vi "Lab Panel V5.26.vi"() -> ()   [LabVIEW 2017] (continued)
              tunnel: w3351 -> [w3361 _ w3422]
              tunnel: w3350 -> [w3359 _ w3421]
              tunnel: w3349 -> [w3360 _ w3420]
              tunnel: w3348 -> [_ w3384 w3419]
              tunnel: w3347 -> [_ w3385 w3418]
              tunnel: w3346 -> [_ w3386 w3417]
              tunnel: w3345 -> [_ w3387 w3416]
              tunnel: w3344 -> [_ w3388 w3415]
              frame #0 {
                n1780 = Select(t=2, s=w3359, f=0) -> (s? t:f=w3355:i32)
                n1781 = Select(t=2, s=w3361, f=0) -> (s? t:f=w3356:i32)
                n1782 = Select(t=2, s=w3360, f=0) -> (s? t:f=w3354:i32)
                n1783 = Select(t=2, s=w3367, f=0) -> (s? t:f=w3358:i32)
                n1784 = Select(t=2, s=w3362, f=0) -> (s? t:f=w3357:i32)
                n1785 = property on="SELECT LAB02-2" class="RadioBtnsControl (strict)"("DisabledEnum"=w3355) -> ()  [unwired: 2 in, 2 out]
                n1786 = property on="SELECT LAB02-1" class="RadioBtnsControl (strict)"("DisabledEnum"=w3356) -> ()  [unwired: 2 in, 2 out]
                n1787 = property on="SELECT LAB03-1" class="RadioBtnsControl (strict)"("DisabledEnum"=w3354) -> ()  [unwired: 2 in, 2 out]
                n1788 = property on="SELECT LAB01-1" class="RadioBtnsControl (strict)"("DisabledEnum"=w3358) -> ()  [unwired: 2 in, 2 out]
                n1789 = property on="SELECT LAB01-2" class="RadioBtnsControl (strict)"("DisabledEnum"=w3357) -> ()  [unwired: 2 in, 2 out]
                n1790 = Not(x=w3367) -> (.not. x?=w3368:bool)
                n1791 = property on="RESULT LAB01-1" class="Bool (strict)"("Visible"=w3368) -> ()  [unwired: 2 in, 2 out]
                n1792 = Not(x=w3362) -> (.not. x?=w3366:bool)
                n1793 = Not(x=w3361) -> (.not. x?=w3365:bool)
                n1794 = Not(x=w3359) -> (.not. x?=w3364:bool)
                n1795 = property on="RESULT LAB01-2" class="Bool (strict)"("Visible"=w3366) -> ()  [unwired: 2 in, 2 out]
                n1796 = Not(x=w3360) -> (.not. x?=w3363:bool)
                n1797 = property on="RESULT LAB02-1" class="Bool (strict)"("Visible"=w3365) -> ()  [unwired: 2 in, 2 out]
                n1798 = property on="RESULT LAB02-2" class="Bool (strict)"("Visible"=w3364) -> ()  [unwired: 2 in, 2 out]
                n1799 = property on="RESULT LAB03-1" class="Bool (strict)"("Visible"=w3363) -> ()  [unwired: 2 in, 2 out]
                n1800 = property on="SET LAB01-1" class="Clust (strict)"("DisabledEnum"=w3358) -> ()  [unwired: 2 in, 2 out]
                n1801 = property on="SET LAB01-2" class="Clust (strict)"("DisabledEnum"=w3357) -> ()  [unwired: 2 in, 2 out]
                n1802 = property on="SET LAB02-1" class="Clust (strict)"("DisabledEnum"=w3356) -> ()  [unwired: 2 in, 2 out]
                n1803 = property on="SET LAB02-2" class="Clust (strict)"("DisabledEnum"=w3355) -> ()  [unwired: 2 in, 2 out]
                n1804 = property on="SET LAB03-1" class="Clust (strict)"("DisabledEnum"=w3354) -> ()  [unwired: 2 in, 2 out]
                n1805 = property on="O/I  LAB01-1" class="Bool (strict)"("DisabledEnum"=w3358) -> ()  [unwired: 2 in, 2 out]
                n1806 = property on="O/I  LAB01-2" class="Bool (strict)"("DisabledEnum"=w3357) -> ()  [unwired: 2 in, 2 out]
                n1807 = property on="O/I  LAB02-1" class="Bool (strict)"("DisabledEnum"=w3356) -> ()  [unwired: 2 in, 2 out]
                n1808 = property on="O/I  LAB02-2" class="Bool (strict)"("DisabledEnum"=w3355) -> ()  [unwired: 2 in, 2 out]
                n1809 = property on="O/I  LAB03-1" class="Bool (strict)"("DisabledEnum"=w3354) -> ()  [unwired: 2 in, 2 out]
              }
              frame #1 {
                n1810 = Select(t=2, s=w3388, f=0) -> (s? t:f=w3379:i32)
                n1811 = Select(t=2, s=w3387, f=0) -> (s? t:f=w3380:i32)
                n1812 = Select(t=2, s=w3384, f=0) -> (s? t:f=w3383:i32)
                n1813 = Select(t=2, s=w3385, f=0) -> (s? t:f=w3382:i32)
                n1814 = Select(t=2, s=w3386, f=0) -> (s? t:f=w3381:i32)
                n1815 = property on="SELECT LAB05-2" class="RadioBtnsControl (strict)"("DisabledEnum"=w3379) -> ()  [unwired: 2 in, 2 out]
                n1816 = property on="SELECT LAB05-1" class="RadioBtnsControl (strict)"("DisabledEnum"=w3380) -> ()  [unwired: 2 in, 2 out]
                n1817 = property on="SELECT LAB03-2" class="RadioBtnsControl (strict)"("DisabledEnum"=w3383) -> ()  [unwired: 2 in, 2 out]
                n1818 = property on="SELECT LAB04-1" class="RadioBtnsControl (strict)"("DisabledEnum"=w3382) -> ()  [unwired: 2 in, 2 out]
                n1819 = property on="SELECT LAB04-2" class="RadioBtnsControl (strict)"("DisabledEnum"=w3381) -> ()  [unwired: 2 in, 2 out]
                n1820 = property on="SET LAB05-2" class="Clust (strict)"("DisabledEnum"=w3379) -> ()  [unwired: 2 in, 2 out]
                n1821 = property on="SET LAB05-1" class="Clust (strict)"("DisabledEnum"=w3380) -> ()  [unwired: 2 in, 2 out]
                n1822 = property on="SET LAB03-2" class="Clust (strict)"("DisabledEnum"=w3383) -> ()  [unwired: 2 in, 2 out]
                n1823 = property on="SET LAB04-1" class="Clust (strict)"("DisabledEnum"=w3382) -> ()  [unwired: 2 in, 2 out]
                n1824 = property on="SET LAB04-2" class="Clust (strict)"("DisabledEnum"=w3381) -> ()  [unwired: 2 in, 2 out]
                n1825 = property on="O/I  LAB05-2" class="Bool (strict)"("DisabledEnum"=w3379) -> ()  [unwired: 2 in, 2 out]
                n1826 = property on="O/I  LAB05-1" class="Bool (strict)"("DisabledEnum"=w3380) -> ()  [unwired: 2 in, 2 out]
                n1827 = property on="O/I  LAB04-1" class="Bool (strict)"("DisabledEnum"=w3382) -> ()  [unwired: 2 in, 2 out]
                n1828 = property on="O/I  LAB04-2" class="Bool (strict)"("DisabledEnum"=w3381) -> ()  [unwired: 2 in, 2 out]
                n1829 = property on="O/I  LAB03-2" class="Bool (strict)"("DisabledEnum"=w3383) -> ()  [unwired: 2 in, 2 out]
                n1830 = Not(x=w3388) -> (.not. x?=w3389:bool)
                n1831 = Not(x=w3387) -> (.not. x?=w3390:bool)
                n1832 = Not(x=w3386) -> (.not. x?=w3391:bool)
                n1833 = property on="RESULT LAB05-2" class="Bool (strict)"("Visible"=w3389) -> ()  [unwired: 2 in, 2 out]
                n1834 = property on="RESULT LAB05-1" class="Bool (strict)"("Visible"=w3390) -> ()  [unwired: 2 in, 2 out]
                n1835 = Not(x=w3385) -> (.not. x?=w3392:bool)
                n1836 = property on="RESULT LAB04-2" class="Bool (strict)"("Visible"=w3391) -> ()  [unwired: 2 in, 2 out]
                n1837 = Not(x=w3384) -> (.not. x?=w3393:bool)
                n1838 = property on="RESULT LAB04-1" class="Bool (strict)"("Visible"=w3392) -> ()  [unwired: 2 in, 2 out]
                n1839 = property on="RESULT LAB03-2" class="Bool (strict)"("Visible"=w3393) -> ()  [unwired: 2 in, 2 out]
              }
              frame #2 {
                # "disable calibrate if any test running"
                n1840 = Or(x=w3416, y=w3415) -> (x .or. y?=w3409:bool)
                n1841 = Or(x=w3418, y=w3417) -> (x .or. y?=w3411:bool)
                n1842 = Or(x=w3422, y=w3421) -> (x .or. y?=w3413:bool)
                n1843 = Or(x=w3420, y=w3419) -> (x .or. y?=w3412:bool)
                n1844 = Or(x=w3424, y=w3423) -> (x .or. y?=w3414:bool)
                n1845 = Or(x=w3412, y=w3411) -> (x .or. y?=w3410:bool)
                n1846 = Or(x=w3414, y=w3413) -> (x .or. y?=w3408:bool)
                n1847 = Or(x=w3410, y=w3409) -> (x .or. y?=w3407:bool)
                n1848 = Or(x=w3408, y=w3407) -> (x .or. y?=w3404:bool)
                "Any Test Running" <- w3404
                n1849 = case shown="False" w3404 {
                  tunnel: [0 2] -> w3406
                  frame False {
                  }
                  frame True {
                  }
                }
                n1850 = property on="JIG TEST" class="Clust (strict)"("DisabledEnum"=w3406) -> ()  [unwired: 2 in, 2 out]
                n1851 = property on="Network Directory" class="Path"("DisabledEnum"=w3406) -> ()  [unwired: 2 in, 2 out]
                n1852 = property on="MAIL SETTINGS" class="Clust (strict)"("DisabledEnum"=w3406) -> ()  [unwired: 2 in, 2 out]
                n1853 = property on="SET (cal)" class="Bool (strict)"("DisabledEnum"=w3406) -> ()  [unwired: 2 in, 2 out]
                n1854 = property on="ADMIN" class="Bool (strict)"("DisabledEnum"=0) -> ()  [unwired: 2 in, 2 out]
              }
            }
          }
          frame #9 {
            # "drive jigs"
            n1855 = stacked-sequence {
              frame #0 {
                # "jig on"
                n1856 = local read "jig cycle"() -> (w3432:dbl)
                n1857 = property on="JIG TEST" class="Clust (strict)"() -> ("DisabledEnum"=w3429:T16)  [unwired: 2 in, 2 out]
                n1858 = Equal?(x=w3429, y=2) -> (x = y?=w3428:bool)
                n1859 = Equal?(x=w3432, y=0) -> (x = y?=w3430:bool)
                n1860 = And(x=w3430, y=w3428) -> (x .and. y?=w3427:bool)
                n1861 = case shown="True" w3427 {
                  frame False {
                  }
                  frame True {
                    n1862 = local read "run lab01-1"() -> (w3443:bool)
                    n1863 = local read "run lab01-2"() -> (w3442:bool)
                    n1864 = local read "run lab02-1"() -> (w3441:bool)
                    n1865 = local read "run lab02-2"() -> (w3440:bool)
                    n1866 = local read "run lab03-1"() -> (w3439:bool)
                    n1867 = local read "run lab03-2"() -> (w3438:bool)
                    n1868 = local read "run lab04-1"() -> (w3437:bool)
                    n1869 = local read "run lab04-2"() -> (w3436:bool)
                    n1870 = local read "run lab05-1"() -> (w3435:bool)
                    n1871 = local read "run lab05-2"() -> (w3434:bool)
                    n1872 = local write "JIG LAB03-2"(w3438) -> ()
                    n1873 = local write "JIG LAB01-1"(w3443) -> ()
                    n1874 = local write "JIG LAB01-2"(w3442) -> ()
                    n1875 = local write "JIG LAB02-1"(w3441) -> ()
                    n1876 = local write "JIG LAB02-2"(w3440) -> ()
                    n1877 = local write "JIG LAB03-1"(w3439) -> ()
                    n1878 = local write "JIG LAB04-1"(w3437) -> ()
                    n1879 = local write "JIG LAB04-2"(w3436) -> ()
                    n1880 = local write "JIG LAB05-1"(w3435) -> ()
                    n1881 = local write "JIG LAB05-2"(w3434) -> ()
                  }
                }
              }
              frame #1 {
                # "jig off"
                n1882 = local read "jig cycle"() -> (w3450:dbl)
                n1883 = local read "on loops"() -> (w3449:dbl)
                n1884 = property on="JIG TEST" class="Clust (strict)"() -> ("DisabledEnum"=w3448:T16)  [unwired: 2 in, 2 out]
                n1885 = Equal?(x=w3448, y=2) -> (x = y?=w3446:bool)
                n1886 = Equal?(x=w3450, y=w3449) -> (x = y?=w3445:bool)
                n1887 = And(x=w3445, y=w3446) -> (x .and. y?=w3444:bool)
                n1888 = case shown="True" w3444 {
                  frame False {
                  }
                  frame True {
                    w3501 = FALSE
                    w3502 = TRUE
                    w3500 = 2
                    n1889 = local read "SELECT LAB05-2"() -> (w3491:T3)
                    n1890 = local read "SELECT LAB04-2"() -> (w3493:T3)
                    n1891 = local read "SELECT LAB04-1"() -> (w3494:T3)
                    n1892 = local read "SELECT LAB05-1"() -> (w3492:T3)
                    n1893 = local read "SELECT LAB03-2"() -> (w3495:T3)
                    n1894 = local read "SELECT LAB02-1"() -> (w3498:T3)
                    n1895 = local read "SELECT LAB03-1"() -> (w3496:T3)
                    n1896 = local read "SELECT LAB02-2"() -> (w3497:T3)
                    n1897 = local read "SELECT LAB01-2"() -> (w3499:T3)
                    n1898 = local read "run lab05-1"() -> (w3461:bool)
                    n1899 = local read "run lab05-2"() -> (w3460:bool)
                    n1900 = local read "run lab04-2"() -> (w3462:bool)
                    n1901 = local read "SELECT LAB01-1"() -> (w3503:T3)
                    n1902 = local read "run lab04-1"() -> (w3463:bool)
                    n1903 = local read "run lab01-1"() -> (w3479:bool)
                    n1904 = local read "run lab01-2"() -> (w3468:bool)
                    n1905 = local read "run lab03-2"() -> (w3464:bool)
                    n1906 = local read "run lab03-1"() -> (w3465:bool)
                    n1907 = local read "run lab02-1"() -> (w3467:bool)
                    n1908 = local read "run lab02-2"() -> (w3466:bool)
                    n1909 = Equal?(x=w3500, y=w3496) -> (x = y?=w3474:bool)
                    n1910 = Equal?(x=w3500, y=w3495) -> (x = y?=w3473:bool)
                    n1911 = Equal?(x=w3500, y=w3494) -> (x = y?=w3472:bool)
                    n1912 = Equal?(x=w3500, y=w3493) -> (x = y?=w3471:bool)
                    n1913 = Equal?(x=w3500, y=w3492) -> (x = y?=w3470:bool)
                    n1914 = Equal?(x=w3500, y=w3491) -> (x = y?=w3469:bool)
                    n1915 = Equal?(x=w3500, y=w3503) -> (x = y?=w3480:bool)
                    n1916 = Equal?(x=w3500, y=w3498) -> (x = y?=w3476:bool)
                    n1917 = Equal?(x=w3500, y=w3497) -> (x = y?=w3475:bool)
                    n1918 = Equal?(x=w3500, y=w3499) -> (x = y?=w3477:bool)
                    n1919 = And(x=w3471, y=w3462) -> (x .and. y?=w3453:bool)
                    n1920 = And(x=w3474, y=w3465) -> (x .and. y?=w3456:bool)
                    n1921 = And(x=w3472, y=w3463) -> (x .and. y?=w3454:bool)
                    n1922 = And(x=w3469, y=w3460) -> (x .and. y?=w3451:bool)
                    n1923 = And(x=w3475, y=w3466) -> (x .and. y?=w3457:bool)
                    n1924 = And(x=w3473, y=w3464) -> (x .and. y?=w3455:bool)
                    n1925 = And(x=w3470, y=w3461) -> (x .and. y?=w3452:bool)
                    n1926 = And(x=w3477, y=w3468) -> (x .and. y?=w3459:bool)
                    n1927 = And(x=w3480, y=w3479) -> (x .and. y?=w3478:bool)
                    n1928 = And(x=w3476, y=w3467) -> (x .and. y?=w3458:bool)
                    n1929 = Select(t=w3502, s=w3478, f=w3501) -> (s? t:f=w3481:bool)
                    n1930 = Select(t=w3502, s=w3459, f=w3501) -> (s? t:f=w3482:bool)
                    n1931 = Select(t=w3502, s=w3458, f=w3501) -> (s? t:f=w3483:bool)
                    n1932 = Select(t=w3502, s=w3457, f=w3501) -> (s? t:f=w3484:bool)
                    n1933 = Select(t=w3502, s=w3456, f=w3501) -> (s? t:f=w3485:bool)
                    n1934 = Select(t=w3502, s=w3455, f=w3501) -> (s? t:f=w3486:bool)
                    n1935 = Select(t=w3502, s=w3454, f=w3501) -> (s? t:f=w3487:bool)
                    n1936 = Select(t=w3502, s=w3453, f=w3501) -> (s? t:f=w3488:bool)
                    n1937 = Select(t=w3502, s=w3452, f=w3501) -> (s? t:f=w3489:bool)
                    n1938 = Select(t=w3502, s=w3451, f=w3501) -> (s? t:f=w3490:bool)
                    n1939 = local write "JIG LAB03-2"(w3486) -> ()
                    n1940 = local write "JIG LAB02-1"(w3483) -> ()
                    n1941 = local write "JIG LAB02-2"(w3484) -> ()
                    n1942 = local write "JIG LAB01-2"(w3482) -> ()
                    n1943 = local write "JIG LAB03-1"(w3485) -> ()
                    n1944 = local write "JIG LAB01-1"(w3481) -> ()
                    n1945 = local write "JIG LAB05-2"(w3490) -> ()
                    n1946 = local write "JIG LAB04-1"(w3487) -> ()
                    n1947 = local write "JIG LAB05-1"(w3489) -> ()
                    n1948 = local write "JIG LAB04-2"(w3488) -> ()
                  }
                }
              }
            }
          }
          frame #10 {
            # "enable  jig test output if no test busy"
            n1949 = property on="JIG TEST" class="Clust (strict)"() -> ("DisabledEnum"=w3506:T16)  [unwired: 2 in, 2 out]
            n1950 = Equal?(x=w3506, y=0) -> (x = y?=w3504:bool)
            n1951 = case shown="True" w3504 {
              frame False {
              }
              frame True {
                n1952 = local read "JIG TEST"() -> (w3517:T10)
                n1953 = Unbundle(w3517) -> ("LAB01-1"=w3516:bool, "LAB01-2"=w3515:bool, "LAB02-1"=w3514:bool, "LAB02-2"=w3513:bool, "LAB03-1"=w3512:bool, "LAB03-2"=w3511:bool, "LAB04-1"=w3510:bool, "LAB04-2"=w3509:bool, "LAB05-1"=w3508:bool, "LAB05-2"=w3507:bool)
                n1954 = local write "JIG LAB05-1"(w3508) -> ()
                n1955 = local write "JIG LAB05-2"(w3507) -> ()
                n1956 = local write "JIG LAB04-1"(w3510) -> ()
                n1957 = local write "JIG LAB04-2"(w3509) -> ()
                n1958 = local write "JIG LAB03-2"(w3511) -> ()
                n1959 = local write "JIG LAB01-1"(w3516) -> ()
                n1960 = local write "JIG LAB02-1"(w3514) -> ()
                n1961 = local write "JIG LAB03-1"(w3512) -> ()
                n1962 = local write "JIG LAB01-2"(w3515) -> ()
                n1963 = local write "JIG LAB02-2"(w3513) -> ()
              }
            }
          }
          frame #11 {
            w3518 = FALSE
            # "Drive digital output and reset USB and temperature network if required."
            n1964 = global read "Global display 3.vi" "cycle O/F"() -> (w3527:bool)
            n1965 = local read "O/I  LAB05-2"() -> (w3520:bool)
            n1966 = local read "O/I  LAB05-1"() -> (w3522:bool)
            n1967 = local read "JIG LAB05-2"() -> (w3519:bool)
            n1968 = local read "O/I  LAB04-2"() -> (w3524:bool)
            n1969 = local read "JIG LAB05-1"() -> (w3521:bool)
            n1970 = local read "JIG LAB04-2"() -> (w3523:bool)
            n1971 = local read "O/I  LAB03-1"() -> (w3538:bool)
            n1972 = local read "O/I  LAB04-1"() -> (w3534:bool)
            n1973 = local read "O/I  LAB02-1"() -> (w3542:bool)
            n1974 = local read "O/I  LAB02-2"() -> (w3540:bool)
            n1975 = local read "O/I  LAB03-2"() -> (w3536:bool)
            n1976 = local read "JIG LAB04-1"() -> (w3533:bool)
            n1977 = local read "JIG LAB03-2"() -> (w3535:bool)
            n1978 = local read "O/I  LAB01-2"() -> (w3544:bool)
            n1979 = local read "JIG LAB02-1"() -> (w3541:bool)
            n1980 = local read "JIG LAB02-2"() -> (w3539:bool)
            n1981 = local read "JIG LAB03-1"() -> (w3537:bool)
            n1982 = local read "O/I  LAB01-1"() -> (w3546:bool)
            n1983 = local read "JIG LAB01-2"() -> (w3543:bool)
            n1984 = local read "JIG LAB01-1"() -> (w3545:bool)
            n1985 = case shown="False" w3527 {
              tunnel: [w3662 FALSE] -> w3526
              frame False {
                n1986 = local read "Analog error"() -> (w3664:bool)
                n1987 = local read "Reset Measuring"() -> (w3663:bool)
                n1988 = Or(x=w3663, y=w3664) -> (x .or. y?=w3662:bool)
              }
              frame True {
              }
            }
            n1989 = Build Array(w3539, w3538, w3537, w3536, w3535, w3534, w3533) -> (w3531:bool[])
            "USB OUT 1" <- w3531
            n1990 = Build Array(w3546, w3545, w3544, w3543, w3542, w3541, w3540) -> (w3532:bool[])
            "USB OUT 0" <- w3532
            n1991 = Build Array(w3524, w3523, w3522, w3521, w3520, w3519, w3518, w3518) -> (w3530:bool[])
            "USB OUT 2" <- w3530
            n1992 = Not(x=w3527) -> (.not. x?=w3528:bool)
            n1993 = local read "Simulate"() -> (w3529:bool)
            n1994 = And(x=w3528, y=w3526) -> (x .and. y?=w3525:bool)
            n1995 = stacked-sequence {
              tunnel: w3532 -> [w3550 w3556]
              tunnel: w3531 -> [w3549 w3555]
              tunnel: w3530 -> [w3548 w3554]
              tunnel: w3529 -> [w3547 w3557]
              tunnel: w3525 -> [_ w3558]
              frame #0 {
                # "drive outputs for normal use"
                n1996 = case shown="False" w3547 {
                  tunnel: w3550 -> [w3553 _]
                  tunnel: w3549 -> [w3552 _]
                  tunnel: w3548 -> [w3551 _]
                  frame False {
                    n1997 = call "sub vi - Drive Relays All v6.vi"("Array #2"=w3551, "Array #1"=w3552, "Array #0"=w3553) -> ()  [unwired: 8 in, 1 out]
                  }
                  frame True {
                  }
                }
              }
              frame #1 {
                # "USB  reset routine"
                n1998 = case shown="True" w3558 {
                  tunnel: w3557 -> [_ w3562]
                  tunnel: w3556 -> [_ w3561]
                  tunnel: w3555 -> [_ w3560]
                  tunnel: w3554 -> [_ w3559]
                  frame False {
                  }
                  frame True {
                    n1999 = stacked-sequence {
                      seq-local: [w3564 _ _ _ _] -> [_ w3570 _ _ _]
                      tunnel: w3562 -> [_ w3574 _ _ _]
                      tunnel: w3561 -> [_ w3573 _ _ _]
                      tunnel: w3560 -> [_ w3572 _ _ _]
                      tunnel: w3559 -> [_ w3571 _ _ _]
                      frame #0 {
                        n2000 = case shown="False" "Auto Reset" {
                          tunnel: [w3567 FALSE] -> w3565
                          frame False {
                            n2001 = Two Button Dialog(message="System reset") -> (T button?=w3567:bool)  [unwired: 2 in]
                          }
                          frame True {
                          }
                        }
                        n2002 = disable-structure shown="Disabled" {
                          frame Disabled {
                            n2003 = local write "Tab Control 2"(5) -> ()
                          }
                          frame Enabled {
                          }
                        }
                        n2004 = Or(x="Auto Reset", y=w3565) -> (x .or. y?=w3564:bool)
                      }
                      frame #1 {
                        n2005 = case shown="True" w3570 {
                          tunnel: w3574 -> [_ w3580]
                          tunnel: w3573 -> [_ w3579]
                          tunnel: w3572 -> [_ w3578]
                          tunnel: w3571 -> [_ w3577]
                          frame False {
                          }
                          frame True {
                            n2006 = stacked-sequence {
                              tunnel: w3580 -> [_ w3598 _]
                              tunnel: bool[] [] -> [w3583 w3597 w3619]
                              tunnel: w3579 -> [_ _ w3618]
                              tunnel: w3578 -> [w3582 _ w3617]
                              tunnel: w3577 -> [w3581 _ w3616]
                              tunnel: 5000 -> [w3584 _ w3615]
                              frame #0 {
                                # "switch off test stations for system reset"
                                n2007 = stacked-sequence {
                                tunnel: w3584 -> [w3588 w3592 w3594]
                                tunnel: w3583 -> [w3587 w3591 w3595]
                                tunnel: w3582 -> [w3586 _ _]
                                tunnel: w3581 -> [w3585 w3590 _]
                                frame #0 {
                                # "drive 1st 7 inputs"
                                n2008 = call "sub vi - Drive Relays All v6.vi"("Array #2"=w3585, "Array #1"=w3586, "Array #0"=w3587) -> ()  [unwired: 8 in, 1 out]
                                n2009 = call "Message Display V1.vi"("Message"="Delay off LAB 01-1 to 02-1", "Delay mS"=w3588) -> ()  [unwired: 10 in]
                                }
                                frame #1 {
                                # "drive 2nd 7 inputs"
                                n2010 = call "sub vi - Drive Relays All v6.vi"("Array #2"=w3590, "Array #1"=w3591, "Array #0"=w3591) -> ()  [unwired: 8 in, 1 out]
                                n2011 = call "Message Display V1.vi"("Message"="Delay off LAB 02-2 to 04-1", "Delay mS"=w3592) -> ()  [unwired: 10 in]
                                }
                                frame #2 {
                                # "drive 3rd 7 inputs"
                                n2012 = call "sub vi - Drive Relays All v6.vi"("Array #2"=w3595, "Array #1"=w3595, "Array #0"=w3595) -> ()  [unwired: 8 in, 1 out]
                                n2013 = call "Message Display V1.vi"("Message"="Delay off LAB 04-2 to 05-2", "Delay mS"=w3594) -> ()  [unwired: 10 in]
                                }
                                }
                              }
                              frame #1 {
                                # "reset all usb modules"
                                n2014 = stacked-sequence {
                                tunnel: w3598 -> [_ w3603]
                                tunnel: w3597 -> [w3601 _]
                                frame #0 {
                                n2015 = local write "AI Task"(FALSE) -> ()
                                n2016 = call "sub vi - Drive Relays All v6.vi"("Array #2"=bool[] [FALSE, FALSE, FALSE, FALSE, FALSE, FALSE, TRUE, FALSE], "Array #1"=w3601, "Array #0"=w3601) -> ()  [unwired: 8 in, 1 out]
                                }
                                frame #1 {
                                n2017 = call "Reset Meas v 5.vi"("simulate"=w3603) -> ("Reset Error"=w3602:bool)  [unwired: 10 in]
                                n2018 = case shown="False" w3602 {
                                frame False {
                                n2019 = local read "AI Task0"() -> (w3610:dbl)
                                n2020 = local read "AI Task1"() -> (w3609:dbl)
                                n2021 = local read "AI Task2"() -> (w3608:dbl)
                                n2022 = local read "RATE (Hz)"() -> (w3607:dbl)
                                n2023 = local read "SAMPLES"() -> (w3606:dbl)
                                n2024 = call "sub vi - AI USB4704 (3)  Create Task v4.vi"(0:w3610, 5:w3609, 7:w3608, "Rate Hz"=w3607, "Samples"=w3606) -> ("TASK USB 0"=w3613:i32, "TASK USB 1"=w3612:i32, "TASK USB 2"=w3611:i32, "AI Task Er"=w3604:bool)  [unwired: 6 in, 1 out]
                                n2025 = local write "AI Task"(TRUE) -> ()
                                n2026 = local write "Reset Error"(w3604) -> ()
                                n2027 = local write "AI Task2"(w3611) -> ()
                                n2028 = local write "AI Task1"(w3612) -> ()
                                n2029 = local write "AI Task0"(w3613) -> ()
                                }
                                frame True {
                                "Reset Error" <- TRUE
                                }
                                }
                                }
                                }
                              }
                              frame #2 {
                                # "switch test stations back on after reset"
                                n2030 = stacked-sequence {
                                tunnel: w3619 -> [w3623 w3626 _]
                                tunnel: w3618 -> [w3622 w3628 w3633]
                                tunnel: w3615 -> [w3621 w3624 w3630]
                                tunnel: w3617 -> [_ w3627 w3632]
                                tunnel: w3616 -> [_ _ w3629]
                                frame #0 {
                                # "drive 1st 7 inputs"
                                n2031 = call "sub vi - Drive Relays All v6.vi"("Array #2"=w3623, "Array #1"=w3623, "Array #0"=w3622) -> ()  [unwired: 8 in, 1 out]
                                n2032 = call "Message Display V1.vi"("Message"="Delay on LAB 01-1 to 02-1", "Delay mS"=w3621) -> ()  [unwired: 10 in]
                                }
                                frame #1 {
                                # "drive 1st & 2nd outputs"
                                n2033 = call "sub vi - Drive Relays All v6.vi"("Array #2"=w3626, "Array #1"=w3627, "Array #0"=w3628) -> ()  [unwired: 8 in, 1 out]
                                n2034 = call "Message Display V1.vi"("Message"="Delay on LAB 02-2 to 04-1", "Delay mS"=w3624) -> ()  [unwired: 10 in]
                                }
                                frame #2 {
                                n2035 = call "sub vi - Drive Relays All v6.vi"("Array #2"=w3629, "Array #1"=w3632, "Array #0"=w3633) -> ()  [unwired: 8 in, 1 out]
                                n2036 = call "Message Display V1.vi"("Message"="Delay on LAB 04-2 to 05-2", "Delay mS"=w3630) -> ()  [unwired: 10 in]
                                }
                                }
                              }
                            }
                          }
                        }
                      }
                      frame #2 {
                        w3634 = 0
                        w3635 = FALSE
                        # "set all back to zero"
                        n2037 = local read "Total USB resets"() -> (w3637:dbl)
                        n2038 = local read "Resets Done"() -> (w3639:dbl)
                        n2039 = local write "Reset Measuring"(w3635) -> ()
                        n2040 = local write "Analog error"(w3635) -> ()
                        n2041 = local write "Er USB#2"(w3634) -> ()
                        n2042 = local write "Er USB#0"(w3634) -> ()
                        n2043 = local write "Er USB#1"(w3634) -> ()
                        n2044 = local write "Error USB #0"(w3635) -> ()
                        n2045 = local write "Error USB #1"(w3635) -> ()
                        n2046 = local write "Error USB #2"(w3635) -> ()
                        n2047 = Increment(x=w3637) -> (x+1=w3636:dbl)
                        n2048 = Increment(x=w3639) -> (x+1=→"Resets Done":dbl)
                        n2049 = local write "Total USB resets"(w3636) -> ()
                      }
                      frame #3 {
                        # "save reset value"
                        n2050 = String To Path(string="c:\\crabtree\\Set Up\\") -> (path=w3649:path)
                        n2051 = Build Path(base path=w3649, name or relative path="USB resets.bin") -> (appended path=w3642:path)
                        n2052 = Create Folder(path (use dialog)=w3649) -> (error out=w3641:errorcluster)  [unwired: 2 in, 2 out]
                        n2053 = local read "Total USB resets"() -> (w3640:dbl)
                        n2054 = call <vilib>:"Clear Errors.vi"("error in (no error)"=w3641) -> ()  [unwired: 5 in, 2 out]
                        n2055 = Open/Create/Replace File(file path (use dialog)=w3642, operation (0:open)=T17."replace or create") -> (refnum out=w3647:refnum<file>, error out=w3646:errorcluster)  [unwired: 4 in, 1 out]
                        n2056 = Write to Binary File(file (use dialog)=w3647, data=w3640, error in=w3646) -> (refnum out=w3645:refnum<file>, error out=w3644:errorcluster)  [unwired: 3 in, 1 out]
                        n2057 = Close File(refnum=w3645, error in=w3644) -> (error out=w3643:errorcluster)  [unwired: 1 out]
                        n2058 = local write "data file error"(w3643) -> ()
                      }
                      frame #4 {
                        # "mail reset value"
                        n2059 = local read "Total USB resets"() -> (w3658:dbl)
                        n2060 = local read "MAIL SETTINGS"() -> (w3654:T7)
                        n2061 = local read "Mail Test File To:"() -> (w3659:string)
                        n2062 = Number To Decimal String(number=w3658) -> (decimal integer string=w3656:string)  [unwired: 1 in]
                        n2063 = Unbundle(w3654) -> ("OUT SERVER ADDRESS"=w3661:string, "FROM ACCOUNT"=w3660:string)  [unwired: 5 out]
                        n2064 = Concatenate Strings("Total USB resets: ", w3656) -> (w3655:string)
                        n2065 = call "Lab Send Mail Test.vi"("TO:"=w3659, "subject"=w3655, "from"=w3660, "out going server"=w3661) -> ("error out"=w3653:errorcluster)  [unwired: 11 in]
                        n2066 = Bundle(cluster=w3654, "mail error"=w3653) -> (w3652:T7)  [unwired: 6 in]
                        n2067 = local write "MAIL SETTINGS"(w3652) -> ()
                      }
                    }
                  }
                }
              }
            }
          }
          frame #12 {
            # "if all test panels are off stop analog read"
            n2068 = local read "O/I  LAB03-1"() -> (w3687:bool)
            n2069 = local read "O/I  LAB03-2"() -> (w3686:bool)
            n2070 = local read "O/I  LAB04-1"() -> (w3685:bool)
            n2071 = local read "O/I  LAB04-2"() -> (w3684:bool)
            n2072 = local read "O/I  LAB05-1"() -> (w3683:bool)
            n2073 = local read "O/I  LAB05-2"() -> (w3682:bool)
            n2074 = local read "O/I  LAB02-2"() -> (w3688:bool)
            n2075 = local read "O/I  LAB02-1"() -> (w3689:bool)
            n2076 = local read "O/I  LAB01-2"() -> (w3690:bool)
            n2077 = local read "O/I  LAB01-1"() -> (w3691:bool)
            n2078 = Or(x=w3683, y=w3682) -> (x .or. y?=w3680:bool)
            n2079 = Or(x=w3685, y=w3684) -> (x .or. y?=w3681:bool)
            n2080 = Or(x=w3689, y=w3688) -> (x .or. y?=w3679:bool)
            n2081 = Or(x=w3687, y=w3686) -> (x .or. y?=w3677:bool)
            n2082 = Or(x=w3691, y=w3690) -> (x .or. y?=w3678:bool)
            n2083 = Or(x=w3681, y=w3680) -> (x .or. y?=w3674:bool)
            n2084 = Or(x=w3678, y=w3679) -> (x .or. y?=w3676:bool)
            n2085 = Or(x=w3676, y=w3677) -> (x .or. y?=w3675:bool)
            n2086 = local read "Any Test Running"() -> (w3673:bool)
            n2087 = Or(x=w3675, y=w3674) -> (x .or. y?=w3672:bool)
            n2088 = local read "AI Task"() -> (w3668:bool)
            n2089 = Or(x=w3672, y=w3673) -> (x .or. y?=w3667:bool)
            n2090 = Not(x=w3667) -> (.not. x?=w3671:bool)
            n2091 = Not(x=w3668) -> (.not. x?=w3669:bool)
            n2092 = And(x=w3671, y=w3668) -> (x .and. y?=w3670:bool)
            n2093 = And(x=w3667, y=w3669) -> (x .and. y?=w3666:bool)
            n2094 = case shown="True" w3670 {
              frame False {
              }
              frame True {
                # "close task if no test"
                n2095 = local read "AI Task2"() -> (w3704:dbl)
                n2096 = local read "AI Task1"() -> (w3703:dbl)
                n2097 = local read "AI Task0"() -> (w3702:dbl)
                n2098 = local write "AI Task"(FALSE) -> ()
                n2099 = call "sub vi - AI USB4704 (3)  Close Task v2.vi"(0:w3702, 5:w3703, 7:w3704) -> ()  [unwired: 13 in]
              }
            }
            n2100 = case shown="True" w3666 {
              frame False {
              }
              frame True {
                # "create task for test"
                n2101 = local read "SAMPLES"() -> (w3696:dbl)
                n2102 = local read "RATE (Hz)"() -> (w3695:dbl)
                n2103 = local read "AI Task2"() -> (w3694:dbl)
                n2104 = local read "AI Task0"() -> (w3692:dbl)
                n2105 = local read "AI Task1"() -> (w3693:dbl)
                n2106 = call "sub vi - AI USB4704 (3)  Create Task v4.vi"(0:w3692, 5:w3693, 7:w3694, "Rate Hz"=w3695, "Samples"=w3696) -> ("TASK USB 0"=w3697:i32, "TASK USB 1"=w3698:i32, "TASK USB 2"=w3699:i32)  [unwired: 6 in, 2 out]
                n2107 = local write "AI Task0"(w3697) -> ()
                n2108 = local write "AI Task1"(w3698) -> ()
                n2109 = local write "AI Task2"(w3699) -> ()
                n2110 = local write "AI Task"(TRUE) -> ()
              }
            }
          }
          frame #13 {
            # "get all analog values from USB devices"
            n2111 = local read "on loops"() -> (w3712:dbl)
            n2112 = local read "jig cycle"() -> (w3709:dbl)
            n2113 = Add(x=w3712, y=3) -> (x+y=w3710:dbl)
            n2114 = Equal?(x=w3709, y=3) -> (x = y?=w3707:bool)
            n2115 = Equal?(x=w3709, y=w3710) -> (x = y?=w3708:bool)
            n2116 = Or(x=w3707, y=w3708) -> (x .or. y?=w3706:bool)
            n2117 = global write "Global display 3.vi" "cycle O/F"(w3707) -> ()
            n2118 = case shown="True" w3706 {
              tunnel: w3707 -> [_ w3718]
              tunnel: w3705 -> [_ w3715]
              frame False {
              }
              frame True {
                n2119 = local read "Simulate"() -> (w3721:bool)
                n2120 = case shown="False" w3721 {
                  tunnel: [w3737 dynamicdata[] [] ("array GRAPH")] -> w3727
                  tunnel: [w3736 w3762] -> w3726
                  tunnel: [w3735 w3762] -> w3725
                  tunnel: [w3734 w3762] -> w3724
                  tunnel: [w3733 w3762] -> w3723
                  tunnel: [w3732 w3762] -> w3722
                  tunnel: w3718 -> [_ w3766]
                  tunnel: [w3731 "Ambient Volts"] -> w3717
                  tunnel: [w3730 bool[] []] -> w3716
                  tunnel: w3715 -> [w3729 _]
                  tunnel: [w3728 0.3 ("Analog loop time")] -> w3714
                  frame False {
                    # "analog in"
                    n2121 = case shown="True" w3729 {
                      tunnel: [dynamicdata[] [] ("array GRAPH") w3756] -> w3737
                      tunnel: [w3739 w3755] -> w3736
                      tunnel: [w3739 w3754] -> w3735
                      tunnel: [w3739 w3753] -> w3734
                      tunnel: [w3739 w3752] -> w3733
                      tunnel: [w3739 w3751] -> w3732
                      tunnel: [3 w3750] -> w3731
                      tunnel: [bool[] [] w3749] -> w3730
                      tunnel: [0.0 w3745] -> w3728
                      frame False {
                        w3740 = 0.0
                        # "no test"
                        n2122 = Bundle(w3740, w3740, w3740, w3740, w3740, w3740) -> (w3739:cluster{dbl, dbl, dbl, dbl, dbl, dbl})  [unwired: 1 in]
                      }
                      frame True {
                        # "test on"
                        n2123 = local read "AI data 0"() -> (w3748:waveform(dbl)[])
                        n2124 = local read "AI data 1"() -> (w3747:waveform(dbl)[])
                        n2125 = local read "AI data 2"() -> (w3744:waveform(dbl)[])
                        n2126 = local read "AI Error"() -> (w3746:errorcluster[])
                        n2127 = call "sub vi - Read Analog All v9.5.vi"("data 0"=w3748, "data 1"=w3747, "data 2"=w3744, "AI Error"=w3746) -> ("array GRAPH"=w3756:dynamicdata[], "LAB01"=w3755:T27, "LAB02"=w3754:T28, "LAB03"=w3753:T29, "LAB04"=w3752:T30, "deg C"=w3750:dbl, "USB Error"=w3749:bool[], "LAB05"=w3751:T31)  [unwired: 4 in]
                        n2128 = local read "AI loop time"() -> (w3745:dbl)
                      }
                    }
                  }
                  frame True {
                    # "simulate"
                    n2129 = local read "ON amps"() -> (w3760:dbl)
                    n2130 = local read "OFF amps"() -> (w3761:dbl)
                    n2131 = local read "VOLTS"() -> (w3764:dbl)
                    n2132 = local read "PF"() -> (w3763:dbl)
                    n2133 = Select(t=w3760, s=w3766, f=w3761) -> (s? t:f=w3765:dbl)
                    n2134 = Bundle("OFF amps"=w3765, "VOLTS"=w3764, "PF"=w3763, "OFF amps"=w3765, "VOLTS"=w3764, "PF"=w3763) -> (w3762:T32)  [unwired: 1 in]
                  }
                }
                n2135 = local read "Simulate"() -> (w3720:bool)
                n2136 = stacked-sequence {
                  seq-local: [w3770 _ _ _ _ _ _ _] -> [_ _ _ _ _ _ _ _]
                  seq-local: [w3769 _ _ _ _ _ _ _] -> [_ _ _ _ _ _ _ _]
                  seq-local: [w3768 _ _ _ _ _ _ _] -> [_ _ _ _ _ _ _ w3963]
                  tunnel: w3727 -> [_ w3821 _ _ _ _ _ _]
                  tunnel: w3726 -> [_ _ w3848 _ _ _ _ _]
                  tunnel: w3725 -> [_ _ _ w3876 _ _ _ _]
                  tunnel: w3724 -> [_ _ _ _ w3904 _ _ _]
                  tunnel: w3723 -> [_ _ _ _ _ w3932 _ _]
                  tunnel: w3722 -> [_ _ _ _ _ _ w3960 _]
                  tunnel: w3720 -> [_ _ w3847 w3875 w3903 w3931 w3959 w3965]
                  tunnel: T14 {"1  (A) cal"=1.0, "1 (V) cal"=1.0, "1 (PF) cal"=1.0, "1 (TL) cal"=1.0, "1 (TN) cal"=1.0, "2 (A) cal"=1.0, "2 (V) cal"=1.0, "2 (PF) cal"=1.0, "2 (TL) cal"=1.0, "2 (TN) cal"=1.0} ("CAL LAB01") -> [_ _ w3846 w3874 w3902 w3930 w3958 _]
                  tunnel: w3717 -> [_ _ _ _ _ _ _ w3964]
                  tunnel: w3716 -> [w3773 _ _ _ _ _ _ _]
                  tunnel: w3714 -> [_ w3800 _ _ _ _ _ _]
                  frame #0 {
                    n2137 = Index Array(array=w3773, index=2) -> (element=w3768:bool)
                    n2138 = Index Array(array=w3773, index=1) -> (element=w3769:bool)
                    n2139 = Index Array(array=w3773, index=0) -> (element=w3770:bool)
                    n2140 = local write "Error USB #2"(w3768) -> ()
                    n2141 = local write "Error USB #0"(w3770) -> ()
                    n2142 = local write "Error USB #1"(w3769) -> ()
                    n2143 = stacked-sequence {
                      tunnel: w3770 -> [w3777 _ _ _]
                      tunnel: w3769 -> [_ w3782 _ _]
                      tunnel: 0 -> [w3776 w3781 w3786 _]
                      tunnel: w3768 -> [_ _ w3787 _]
                      frame #0 {
                        n2144 = case shown="True" w3777 {
                          tunnel: w3776 -> [w3778 _]
                          frame False {
                            n2145 = local write "Er USB#0"(w3778) -> ()
                          }
                          frame True {
                            n2146 = local read "Er USB#0"() -> (w3780:dbl)
                            n2147 = Increment(x=w3780) -> (x+1=→"Er USB#0":dbl)
                          }
                        }
                      }
                      frame #1 {
                        n2148 = case shown="True" w3782 {
                          tunnel: w3781 -> [w3783 _]
                          frame False {
                            n2149 = local write "Er USB#1"(w3783) -> ()
                          }
                          frame True {
                            n2150 = local read "Er USB#1"() -> (w3785:dbl)
                            n2151 = Increment(x=w3785) -> (x+1=→"Er USB#1":dbl)
                          }
                        }
                      }
                      frame #2 {
                        n2152 = case shown="True" w3787 {
                          tunnel: w3786 -> [w3788 _]
                          frame False {
                            n2153 = local write "Er USB#2"(w3788) -> ()
                          }
                          frame True {
                            n2154 = local read "Er USB#2"() -> (w3790:dbl)
                            n2155 = Increment(x=w3790) -> (x+1=→"Er USB#2":dbl)
                          }
                        }
                      }
                      frame #3 {
                        w3796 = 10
                        n2156 = local read "Er USB#2"() -> (w3797:dbl)
                        n2157 = local read "Er USB#0"() -> (w3799:dbl)
                        n2158 = local read "Er USB#1"() -> (w3798:dbl)
                        n2159 = Greater Or Equal?(x=w3799, y=w3796) -> (x >= y?=w3794:bool)
                        n2160 = Greater Or Equal?(x=w3798, y=w3796) -> (x >= y?=w3793:bool)
                        n2161 = Greater Or Equal?(x=w3797, y=w3796) -> (x >= y?=w3792:bool)
                        n2162 = Or(x=w3794, y=w3793) -> (x .or. y?=w3795:bool)
                        n2163 = Or(x=w3795, y=w3792) -> (x .or. y?=→"Analog error":bool)
                      }
                    }
                  }
                  frame #1 {
                    # "display graph data on ADM page"
                    n2164 = local write "AI loop time"(w3800) -> ()
                    n2165 = local write "AI"(TRUE) -> ()
                    n2166 = Index Array(array=w3821, index=6) -> (element=→"LAB04-1 (GRAPH)":dynamicdata)
                    n2167 = Index Array(array=w3821, index=7) -> (element=→"LAB04-2 (GRAPH)":dynamicdata)
                    n2168 = Index Array(array=w3821, index=9) -> (element=→"LAB05-2 (GRAPH)":dynamicdata)
                    n2169 = Index Array(array=w3821, index=8) -> (element=→"LAB05-1 (GRAPH)":dynamicdata)
                    n2170 = Index Array(array=w3821, index=5) -> (element=→"LAB03-2 (GRAPH)":dynamicdata)
                    n2171 = Index Array(array=w3821, index=0) -> (element=→"LAB01-1 (GRAPH)":dynamicdata)
                    n2172 = Index Array(array=w3821, index=1) -> (element=→"LAB01-2 (GRAPH)":dynamicdata)
                    n2173 = Index Array(array=w3821, index=2) -> (element=→"LAB02-1 (GRAPH)":dynamicdata)
                    n2174 = Index Array(array=w3821, index=3) -> (element=→"LAB02-2 (GRAPH)":dynamicdata)
                    n2175 = Index Array(array=w3821, index=4) -> (element=→"LAB03-1 (GRAPH)":dynamicdata)
                  }
                  frame #2 {
                    n2176 = case shown="False" w3847 {
                      tunnel: [w3849 w3850] -> w3845
                      tunnel: w3846 -> [_ w3850]
                      frame False {
                        n2177 = local read "CAL LAB01"() -> (w3849:T14)
                      }
                      frame True {
                      }
                    }
                    n2178 = Unbundle By Name(w3848) -> ("OFF amps"=w3844:dbl, "VOLTS"=w3843:dbl, "PF"=w3842:dbl, "OFF amps"=w3841:dbl, "VOLTS"=w3840:dbl, "PF"=w3839:dbl)
                    n2179 = Unbundle By Name(w3845) -> ("1  (A) cal"=w3838:dbl, "1 (V) cal"=w3837:dbl, "1 (PF) cal"=w3836:dbl, "2 (A) cal"=w3835:dbl, "2 (V) cal"=w3834:dbl, "2 (PF) cal"=w3833:dbl)  [unwired: 4 out]
                    n2180 = Multiply(x=w3844, y=w3838) -> (x*y=w3831:dbl)
                    n2181 = Multiply(x=w3843, y=w3837) -> (x*y=w3830:dbl)
                    n2182 = Multiply(x=w3842, y=w3836) -> (x*y=w3829:dbl)
                    n2183 = Multiply(x=w3841, y=w3835) -> (x*y=w3827:dbl)
                    n2184 = Multiply(x=w3840, y=w3834) -> (x*y=w3826:dbl)
                    n2185 = Multiply(x=w3839, y=w3833) -> (x*y=w3825:dbl)
                    n2186 = local read "SIG LAB01-1"() -> (w3832:T2)
                    n2187 = local read "SIG LAB01-2"() -> (w3828:T2)
                    n2188 = Bundle By Name(cluster=w3832, "AMPS"=w3831, "VOLTS"=w3830, "PF"=w3829) -> (w3824:T2)
                    n2189 = Bundle By Name(cluster=w3828, "AMPS"=w3827, "VOLTS"=w3826, "PF"=w3825) -> (w3823:T2)
                    n2190 = global write "Global display 1.vi" "SIG LAB01-2"(w3823) -> ()
                    n2191 = global write "Global display 1.vi" "SIG LAB01-1"(w3824) -> ()
                    n2192 = local write "SIG LAB01-2"(w3823) -> ()
                    n2193 = local write "SIG LAB01-1"(w3824) -> ()
                  }
                  frame #3 {
                    n2194 = Unbundle By Name(w3876) -> ("OFF amps"=w3872:dbl, "VOLTS"=w3871:dbl, "PF"=w3870:dbl, "OFF amps"=w3869:dbl, "VOLTS"=w3868:dbl, "PF"=w3867:dbl)
                    n2195 = case shown="True" w3875 {
                      tunnel: [w3877 w3878] -> w3873
                      tunnel: w3874 -> [_ w3878]
                      frame False {
                        n2196 = local read "CAL LAB02"() -> (w3877:T15)
                      }
                      frame True {
                      }
                    }
                    n2197 = Unbundle By Name(w3873) -> ("1  (A) cal"=w3866:dbl, "1 (V) cal"=w3865:dbl, "1 (PF) cal"=w3864:dbl, "2 (A) cal"=w3863:dbl, "2 (V) cal"=w3862:dbl, "2 (PF) cal"=w3861:dbl)  [unwired: 4 out]
                    n2198 = Multiply(x=w3872, y=w3866) -> (x*y=w3859:dbl)
                    n2199 = Multiply(x=w3871, y=w3865) -> (x*y=w3858:dbl)
                    n2200 = Multiply(x=w3870, y=w3864) -> (x*y=w3857:dbl)
                    n2201 = Multiply(x=w3869, y=w3863) -> (x*y=w3855:dbl)
                    n2202 = Multiply(x=w3868, y=w3862) -> (x*y=w3854:dbl)
                    n2203 = Multiply(x=w3867, y=w3861) -> (x*y=w3853:dbl)
                    n2204 = local read "SIG LAB02-1"() -> (w3860:T2)
                    n2205 = local read "SIG LAB02-2"() -> (w3856:T2)
                    n2206 = Bundle By Name(cluster=w3860, "AMPS"=w3859, "VOLTS"=w3858, "PF"=w3857) -> (w3852:T2)
                    n2207 = Bundle By Name(cluster=w3856, "AMPS"=w3855, "VOLTS"=w3854, "PF"=w3853) -> (w3851:T2)
                    n2208 = global write "Global display 1.vi" "SIG LAB02-1"(w3852) -> ()
                    n2209 = local write "SIG LAB02-2"(w3851) -> ()
                    n2210 = global write "Global display 1.vi" "SIG LAB02-2"(w3851) -> ()
                    n2211 = local write "SIG LAB02-1"(w3852) -> ()
                  }
                  frame #4 {
                    n2212 = Unbundle By Name(w3904) -> ("OFF amps"=w3900:dbl, "VOLTS"=w3899:dbl, "PF"=w3898:dbl, "OFF amps"=w3897:dbl, "VOLTS"=w3896:dbl, "PF"=w3895:dbl)
                    n2213 = case shown="True" w3903 {
                      tunnel: [w3905 w3906] -> w3901
                      tunnel: w3902 -> [_ w3906]
                      frame False {
                        n2214 = local read "CAL LAB03"() -> (w3905:T14)
                      }
                      frame True {
                      }
                    }
                    n2215 = Unbundle By Name(w3901) -> ("1  (A) cal"=w3894:dbl, "1 (V) cal"=w3893:dbl, "1 (PF) cal"=w3892:dbl, "2 (A) cal"=w3891:dbl, "2 (V) cal"=w3890:dbl, "2 (PF) cal"=w3889:dbl)  [unwired: 4 out]
                    n2216 = Multiply(x=w3900, y=w3894) -> (x*y=w3887:dbl)
